vi "Main.vi"() -> ()   [LabVIEW 2013, in "User Event Collection.lvclass"]
uses:
  User Event Collection.lvclass
  Method/Tag.ctl
panel:
  in  "停止":bool
  out "数据":variant
  out "Name":string
  in  "Main":dbl
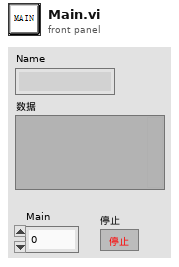
[diagram p1: front panel]
types:
  T1 = enum16{"Init", "Post Event", "Destroy", "Reg Ref"}
  T2 = typedef "User Event Collection.lvclass/Tag.ctl" = enum16{"Main", "UI"}
  T3 = typedef "NISAST Event.lvclass/Event Registeration Refnum.ctl" = refnum<event-registration>
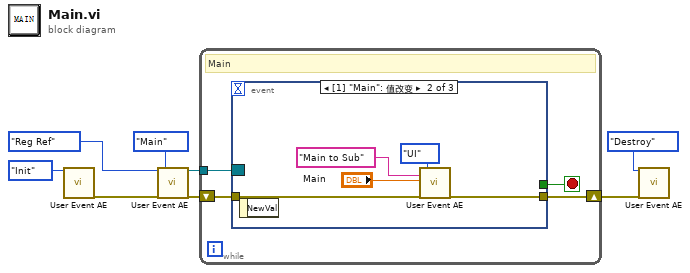
[diagram p0: block diagram]
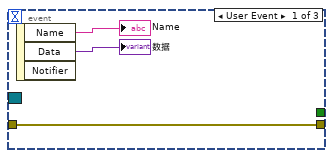
[diagram p2: hidden frame]
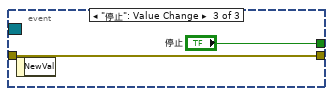
[diagram p3: hidden frame]
diagram:
  n1 = call "User Event AE.vi"("Mode"=T1."Init") -> ("error out"=w7:errorcluster)  [unwired: 17 in, 1 out]
  n2 = call "User Event AE.vi"("Mode"=T1."Reg Ref", "error in (no error)"=w7, "Tag"=Tag."Main") -> ("Event Registration Refnum"=w4:T3, "error out"=w1:errorcluster)  [unwired: 15 in]
  n3 = while {
    tunnel: w4 -> [w12]
    shift-right: [w9] -> w3
    shift-left: w1 -> [w10]
    stop <- w11 stop-if-true
    # "Main"
    n4 = event shown="[1] \"Main\": 值改变" {
      selector: w12 -> [_ _ _]
      dyn-events: _ -> [_ _ _]
      timeout: _ -> [_ _ _]
      tunnel: [_ _ "停止"] -> w11
      tunnel: w10 -> [w13 w17 w21]
      tunnel: [w13 w16 w21] -> w9
      event User Event {
        n5 = event-data() -> ("Name"=→"Name":string, "Data"=→"数据":variant)  [unwired: 1 in, 1 out]
      }
      event "Main": Value Change {
        n6 = event-data() -> ()  [unwired: 1 in, 1 out]
        n7 = call "User Event AE.vi"("Event Name"="Main to Sub", "Event Data"="Main", "error in (no error)"=w17, "Tag"=Tag."UI") -> ("error out"=w16:errorcluster)  [unwired: 14 in, 1 out]
      }
      event "停止": Value Change {
        n8 = event-data() -> ()  [unwired: 1 in, 1 out]
      }
    }
  }
  n9 = call "User Event AE.vi"("Mode"=T1."Destroy", "error in (no error)"=w3) -> ()  [unwired: 16 in, 2 out]
